vi "Assert String Ends With.vi"(4 "Execution time (s)":dbl=-1.0, 5 "Assert Only? (F)":bool, 6 "error code (1)":i32=1, 7 "Label (\"\")":string, 8 "error in (no error)":errorcluster, 9 "Register with caller test (F)":bool, 10 "Substring":string, 11 "String":string) -> (0 "error out":errorcluster, 2 "Properties.Assert":refnum<class "Properties.Assert.lvclass">)   [LabVIEW 2013, in "Caraya.lvlib" / "Assert.lvclass"]
doc: "Asserts that a string ends with a substring."
uses:
  Assert.lvclass
  Properties.Assert/Properties.Assert.lvclass
  Properties/Properties.lvclass
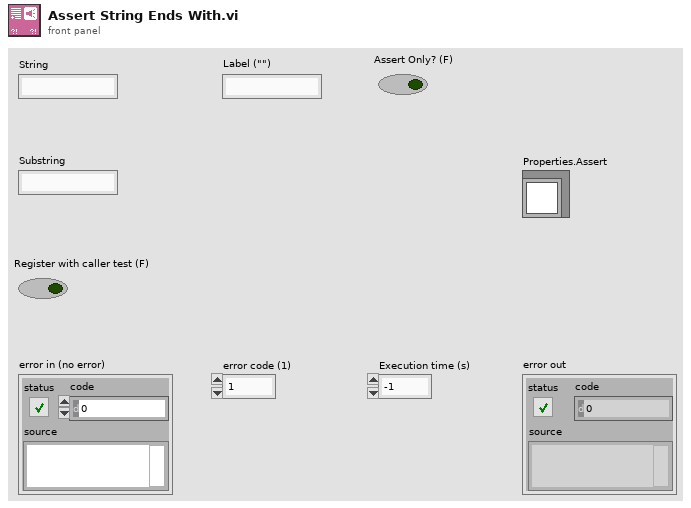
[diagram p1: front panel]
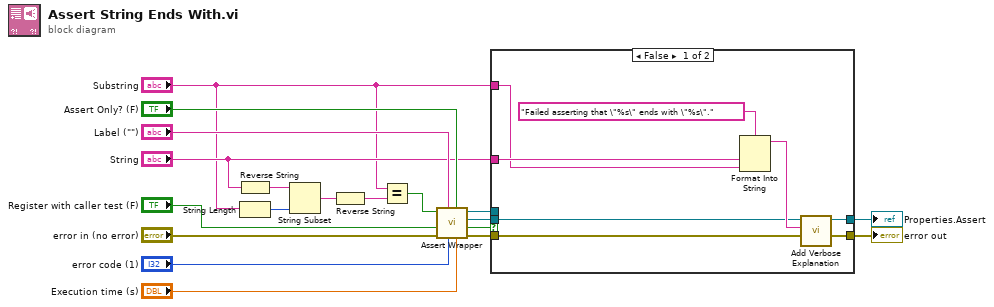
[diagram p0: block diagram]
diagram:
  n1 = Reverse String(1:"String") -> (0:w6:string)
  n2 = String Length(string="Substring") -> (length=w1:i32)
  n3 = String Subset(string=w6, length (rest)=w1) -> (substring=w5:string)  [unwired: 1 in]
  n4 = Reverse String(1:w5) -> (0:w4:string)
  n5 = Equal?(x="Substring", y=w4) -> (x = y?=w2:bool)
  n6 = call "Assert Wrapper.vi"("Execution time (s)"="Execution time (s)", "Assert Only? (F)"="Assert Only? (F)", "error code (1)"="error code (1)", "Label"="Label (\"\")", "error in (no error)"="error in (no error)", "Register with caller test (F)"="Register with caller test (F)", "Assert?"=w2) -> ("error out"=w9:errorcluster, "Verbose"=w13:bool, "Properties.Assert"=w11:refnum<class "Properties.Assert.lvclass">, "Assert out"=w12:refnum<class "Assert.lvclass">)  [unwired: 1 in]
  n7 = case shown="False" w13 {
    tunnel: w12 -> [_ _]
    tunnel: w11 -> [w22 w29]
    tunnel: [w24 w28] -> w10
    tunnel: w9 -> [w25 w28]
    tunnel: "Substring" -> [w26 _]
    tunnel: "String" -> [w27 _]
    tunnel: [w21 w29] -> w8
    frame False {
      n8 = Format Into String(format string="Failed asserting that \"%s\" ends with \"%s\".", w27, w26) -> (resulting string=w23:string)  [unwired: 2 in, 1 out]
      n9 = call "Add Verbose Explanation.vi"("error in (no error)"=w25, "Verbose Explanation"=w23, "Properties"=w22) -> ("error out"=w24:errorcluster, "Properties"=w21:refnum<class "Properties.Assert.lvclass">)  [unwired: 7 in]
    }
    frame True {
    }
  }
  "error out" <- w10
  "Properties.Assert" <- w8
